vi "Image_Actions_V2.vi"(0 "Image Pixel Size Array":T1(array[cluster]), 2 "Mode":u16(ring) items=["Write", "Read"], 7 "Number of Channels":i32, 11 "Action":string) -> (4 "Image REFs OUT":T2[](array[typedef]), 15 "Image Names OUT":string[](array[string]))   [LabVIEW 2016]
uses:
  <vilib>/vision/Image Controls.llb/IMAQ Image.ctl
panel:
  # "Copyright (C) 2020 Edward S Allgeyer\n\nRedistribution and use in source and binary forms, with or without\nmodification, are permitted provided that the following conditions\nare met:\n\n1. Redistributions of source code must retain the above copyright\n   notice, this list of conditions and the following disclaimer.\n\n2. Redistributions in binary form must reproduce the above copyright\n   notice, this list of conditions and the following disclaimer in\n   the documentation and/or other materials provided with the\n   distribution.\n\n3. Neither the name of the copyright holder nor the names of its\n   contributors may be used to endorse or promote products derived\n   from this software without specific prior written permission.\n\nTHIS SOFTWARE IS PROVIDED BY THE COPYRIGHT HOLDERS AND CONTRIBUTORS\n\"AS IS\" AND ANY EXPRESS OR IMPLIED WARRANTIES, INCLUDING, BUT NOT\nLIMITED TO, THE IMPLIED WARRANTIES OF MERCHANTABILITY AND FITNESS\nFOR A PARTICULAR PURPOSE ARE DISCLAIMED. IN NO EVENT SHALL THE\nCOPYRIGHT HOLDER OR CONTRIBUTORS BE LIABLE FOR ANY DIRECT, INDIRECT,\nINCIDENTAL, SPECIAL, EXEMPLARY, OR CONSEQUENTIAL DAMAGES (INCLUDING,\nBUT NOT LIMITED TO, PROCUREMENT OF SUBSTITUTE GOODS OR SERVICES;\nLOSS OF USE, DATA, OR PROFITS; OR BUSINESS INTERRUPTION) HOWEVER\nCAUSED AND ON ANY THEORY OF LIABILITY, WHETHER IN CONTRACT, STRICT\nLIABILITY, OR TORT (INCLUDING NEGLIGENCE OR OTHERWISE) ARISING IN\nANY WAY OUT OF THE USE OF THIS SOFTWARE, EVEN IF ADVISED OF THE\nPOSSIBILITY OF SUCH DAMAGE."
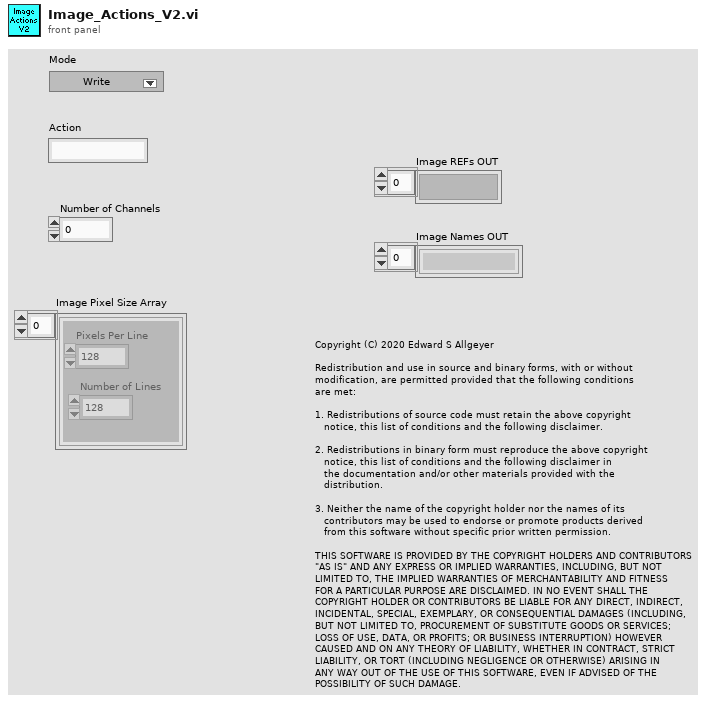
[diagram p1: front panel]
types:
  T1 = cluster{"Pixels Per Line":i32, "Number of Lines":i32}[]
  T2 = typedef "IMAQ Image.ctl" = refnum<image>
  T3 = typedef "Image Type" = u32
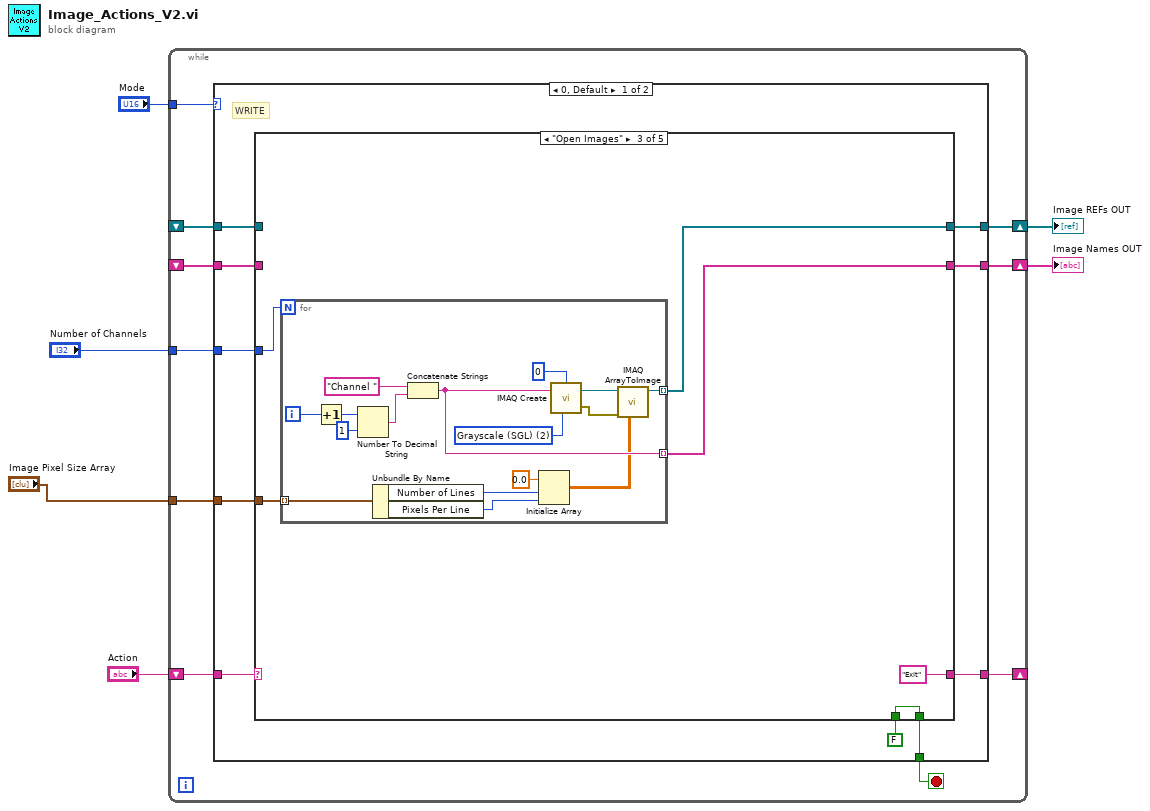
[diagram p0: block diagram]
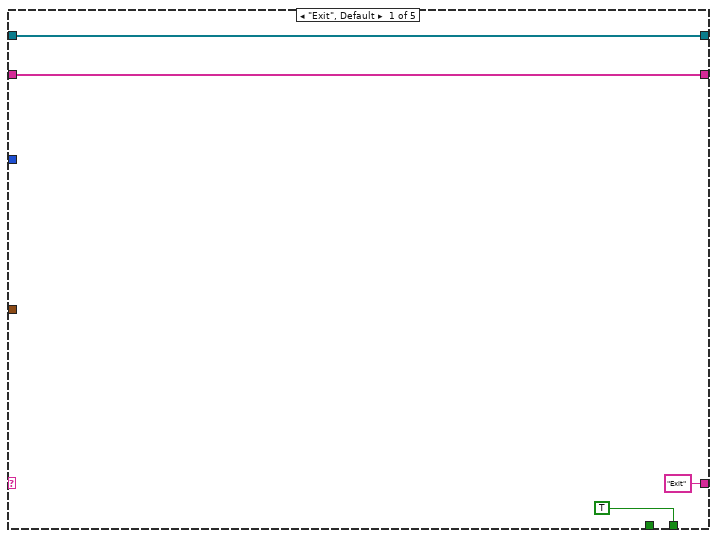
[diagram p2: hidden frame]
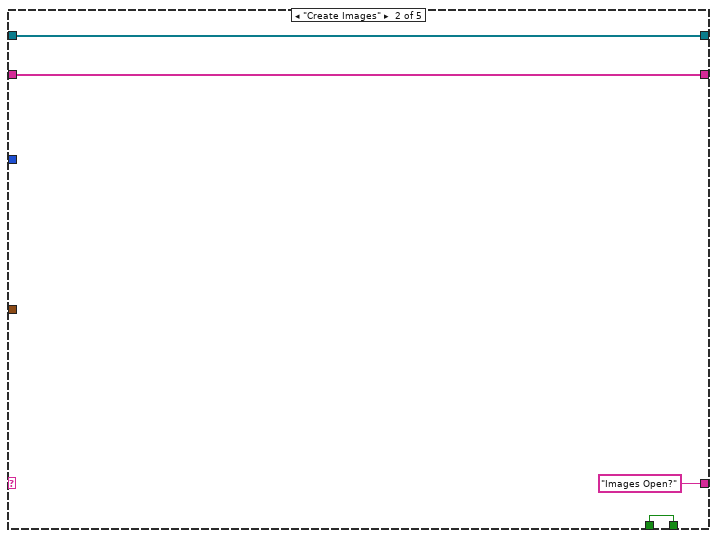
[diagram p3: hidden frame]
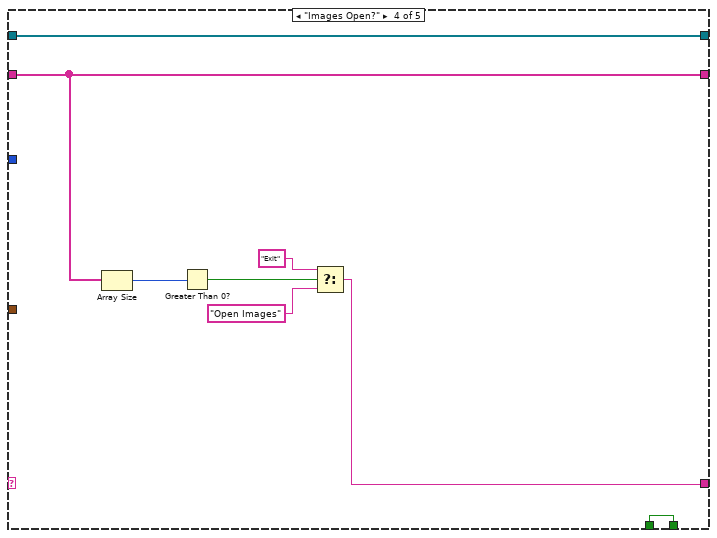
[diagram p4: hidden frame]
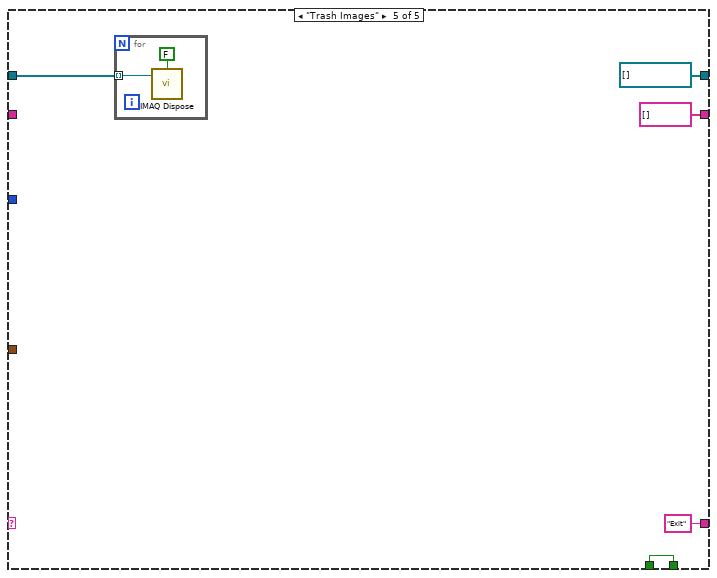
[diagram p5: hidden frame]
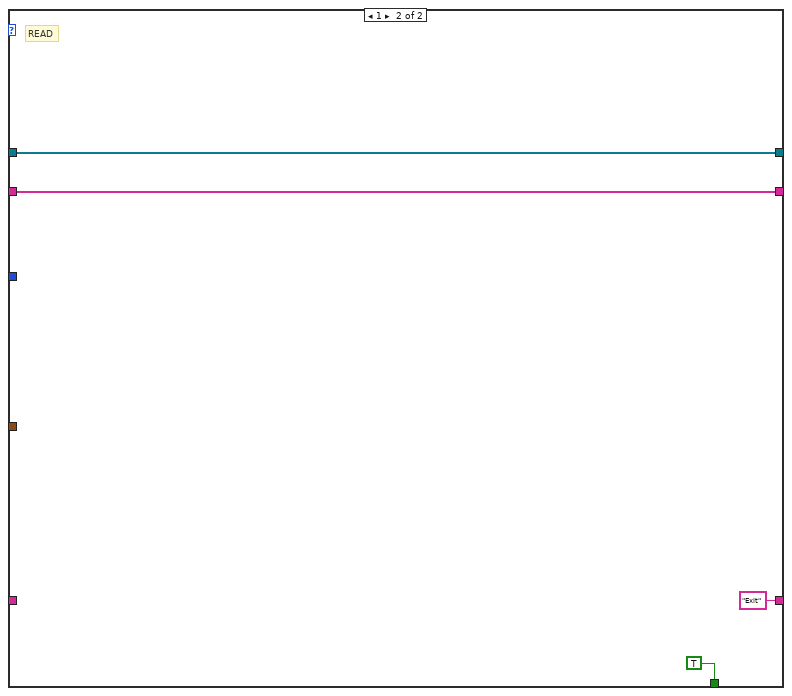
[diagram p6: hidden frame]
diagram:
  n1 = while {
    tunnel: "Mode" -> [w16]
    shift-right: [w7] -> _
    shift-left: "Action" -> [w14]
    shift-right: [w11] -> w3
    shift-left: _ -> [w9]
    tunnel: "Number of Channels" -> [w13]
    tunnel: "Image Pixel Size Array" -> [w12]
    shift-right: [w10] -> w2
    shift-left: _ -> [w8]
    stop <- w15 stop-if-true
    n2 = case shown="0, Default" w16 {
      tunnel: [w21 TRUE] -> w15
      tunnel: w14 -> [w26 _]
      tunnel: w13 -> [w25 _]
      tunnel: w12 -> [w24 _]
      tunnel: [w23 w74] -> w11
      tunnel: [w22 w73] -> w10
      tunnel: w9 -> [w18 w74]
      tunnel: w8 -> [w17 w73]
      tunnel: [w19 "Exit"] -> w7
      frame 0, Default {
        # "WRITE"
        n3 = case shown="\"Open Images\"" w26 {
          tunnel: w25 -> [_ _ w40 _ _]
          tunnel: w24 -> [_ _ w35 _ _]
          tunnel: [w28 w32 w39 w63 T2[] []] -> w23
          tunnel: [w27 w31 w38 w62 string[] []] -> w22
          tunnel: [TRUE w34 w37 w64 w67] -> w21
          tunnel: FALSE -> [_ w34 w37 w64 w67]
          tunnel: ["Exit" "Images Open?" "Exit" w59 "Exit"] -> w19
          tunnel: w18 -> [w28 w32 _ w63 w65]
          tunnel: w17 -> [w27 w31 _ w62 _]
          frame "Exit", Default {
          }
          frame "Create Images" {
          }
          frame "Open Images" {
            n4 = for {
              N: w40 -> [_]
              tunnel: [w47] -> w39 mode=indexing
              tunnel: [w46] -> w38 mode=indexing
              tunnel: w35 -> [w41] mode=indexing
              i -> [w48]
              w52 = T3 2 items=["Grayscale (U8)", "Grayscale (I16)", "Grayscale (SGL)", "Complex (CSG)", "RGB (U32)", "HSL (U32)", "RGB (U64)", "Grayscale (U16)"] ("Image Type")
              n5 = Increment(x=w48) -> (x+1=w54:i32)
              n6 = Number To Decimal String(number=w54, width (-)=i16 1) -> (decimal integer string=w51:string)
              n7 = Unbundle By Name(w41) -> ("Number of Lines"=w44:i32, "Pixels Per Line"=w43:i32)
              n8 = Concatenate Strings("Channel ", w51) -> (w46:string)
              n9 = Initialize Array(sgl 0.0 ("element"), w44, w43) -> (w42:sgl[][])
              n10 = call "IMAQ Create"("Border Size"=0, "Image Name"=w46, "Image Type"=w52) -> ("New Image"=w53:T2, "error out"=w56:errorcluster)  [unwired: 2 in]
              n11 = call "IMAQ ArrayToImage"("Image Pixels (Float)"=w42, "error in (no error)"=w56, "Image"=w53) -> ("Image Out"=w47:T2)  [unwired: 7 in, 1 out]
            }
          }
          frame "Images Open?" {
            n12 = Array Size(array=w62) -> (size(s)=w61:i32)
            n13 = Greater Than 0?(x=w61) -> (x > 0?=w60:bool)
            n14 = Select(t="Exit", s=w60, f="Open Images") -> (s? t:f=w59:string)
          }
          frame "Trash Images" {
            n15 = for {
              tunnel: w65 -> [w71] mode=indexing
              n16 = call "IMAQ Dispose"("All Images? (No)"=FALSE, "Image"=w71) -> ()  [unwired: 4 in, 1 out]
            }
          }
        }
      }
      frame 1 {
        # "READ"
      }
    }
  }
  "Image REFs OUT" <- w3
  "Image Names OUT" <- w2
